vi "HMI.vi"(8 "error in (no error)":errorcluster caption="entrée d'erreur (pas d'erreur)", 11 "Class Popup Autotest (Default) en entrée":refnum<class "Popup Autotest_With_Actor.lvclass">) -> (0 "error out":errorcluster caption="sortie d'erreur", 1 "Input":string, 2 "Autotest":bool, 3 "Class Popup Autotest (Default) en sortie":refnum<class "Popup Autotest_With_Actor.lvclass">)   [LabVIEW 2020, in "Library Instrument & Equipement.lvlib" / "Library Popup.lvlib" / "Popup Autotest_With_Actor.lvclass"]
uses:
  Popup Autotest_With_Actor.lvclass
  C:/Users/ngarcin/OneDrive - Altyor/Standard TB/Class/Popup/Class Popup (Main)/Class Popup (Main).lvclass
  C:/Users/ngarcin/OneDrive - Altyor/Standard TB/Class/Popup/Class Popup Autotest (Default)/Popup Autotest (Default).lvclass
  Commun VI/TypeDef/Commande Popup autotest/Commande element autotest.ctl
  Instrument/Instrument (Default)/Class Instrument (Default).lvclass
  Core/Actors/Actor_Autotest/Auto-test/Auto-test/Actor_Autotest.lvclass
  C:/Program Files (x86)/National Instruments/LabVIEW 2020/vi.lib/ActorFramework/Actor/Actor.lvclass
  Core/Actors/Actor_Autotest/Auto-test/Actor_Autotest Messages/Load_Instr_Object Msg/Load_Instr_Object Msg.lvclass/Load_Instr_Object Msg.ctl
  <vilib>/ActorFramework/Message Enqueuer/Message Enqueuer.lvclass/Message Enqueuer.ctl
  <vilib>/ActorFramework/Stop Msg/Stop Msg.lvclass/Stop Msg.ctl
  <vilib>/ActorFramework/Message Enqueuer/Enqueue.vi
  <vilib>/ActorFramework/Message Enqueuer/Enqueue Critical.vi
  Core/Actors/Actor_Autotest/Auto-test/Actor_Autotest Messages/Load_Instr_Object Msg/Load_Instr_Object Msg.lvclass
  C:/Program Files (x86)/National Instruments/LabVIEW 2020/vi.lib/ActorFramework/Message/Message.lvclass
  Core/Actors/Actor_Autotest/Auto-test/Actor_Autotest Messages/Register_Actor Msg/Register_Actor Msg.lvclass
  <vilib>/ActorFramework/Stop Msg/Stop Msg.lvclass
  <vilib>/ActorFramework/Message Priority Queue/Priority Enqueue.vi
  Variable Instr.vi
  <vilib>/regexp/Match Regular Expression.xnode
  Class Popup Autotest (Default)/Popup Autotest (Default).lvclass
  Popup Autotest_With_Actor.lvclass/Popup Autotest_With_Actor.ctl
  <vilib>/ActorFramework/Actor/Actor.lvclass
  Commun VI/Library Commun.lvlib
panel:
  out "Element test":T2
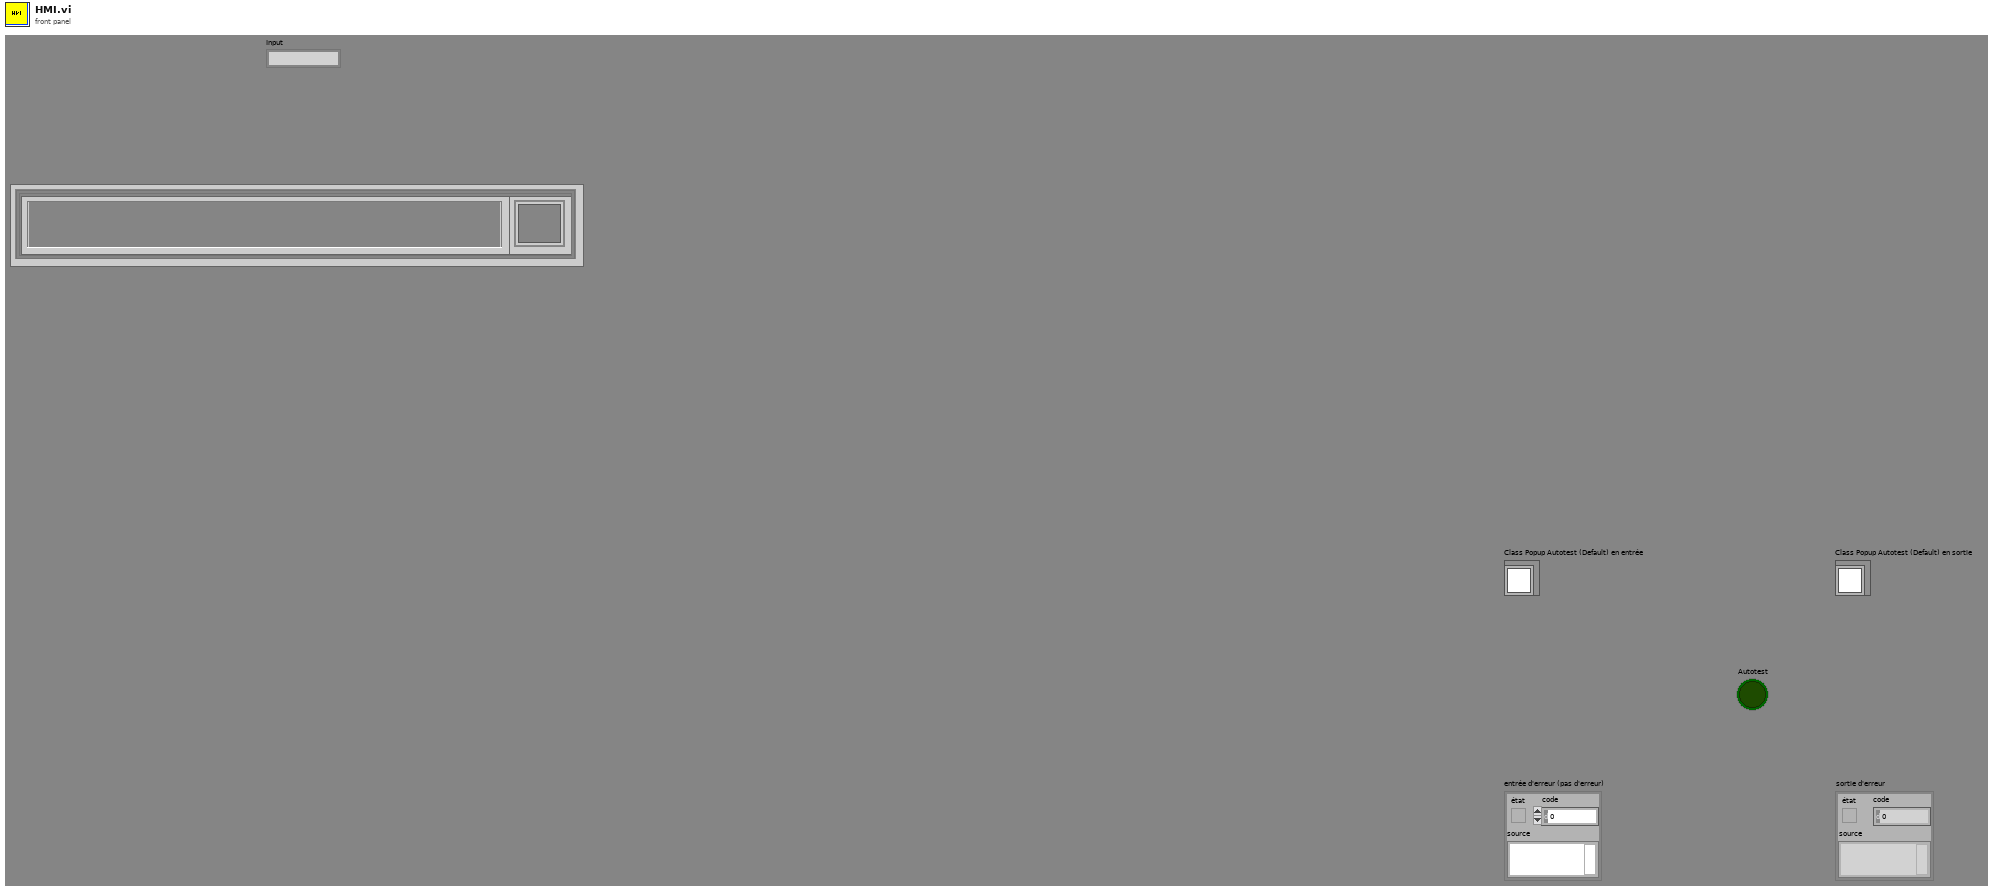
[diagram p1: front panel]
types:
  T1 = typedef "Commande element autotest.ctl" = cluster{"Instrument":string, "Etat":cluster{"Menu déroulant":u16}}
  T2 = cluster{"Element autotest":T1, "Element autotest 2":T1, "Element autotest 3":T1, "Element autotest 4":T1, "Element autotest 5":T1, "Element autotest 6":T1, "Element autotest 7":T1, "Element autotest 8":T1, "Element autotest 9":T1}
  T3 = cluster{"Instrument":refnum<class "Class Instrument (Default).lvclass">, "Element autotest":T1}
  T4 = cluster{"Name":string, "Instrument":refnum<class "Class Instrument (Default).lvclass">, "Close After Autotest":bool}[]
  T5 = enum16{"Init", "Add Actor", "Delete Actor", "Get Actor Queue", "Get Log Actor Queue", "List all actors"}
  T6 = cluster{"Name":string, "Instrument":refnum<class "Class Instrument (Default).lvclass">, "Close After Autotest":bool}
  T7 = cluster{"[0]":T1, "[1]":T1, "[2]":T1, "[3]":T1, "[4]":T1, "[5]":T1, "[6]":T1, "[7]":T1, "[8]":T1}
  T8 = typedef "LVRectTypeDef.ctl" = cluster{"Left":i16, "Top":i16, "Right":i16, "Bottom":i16}
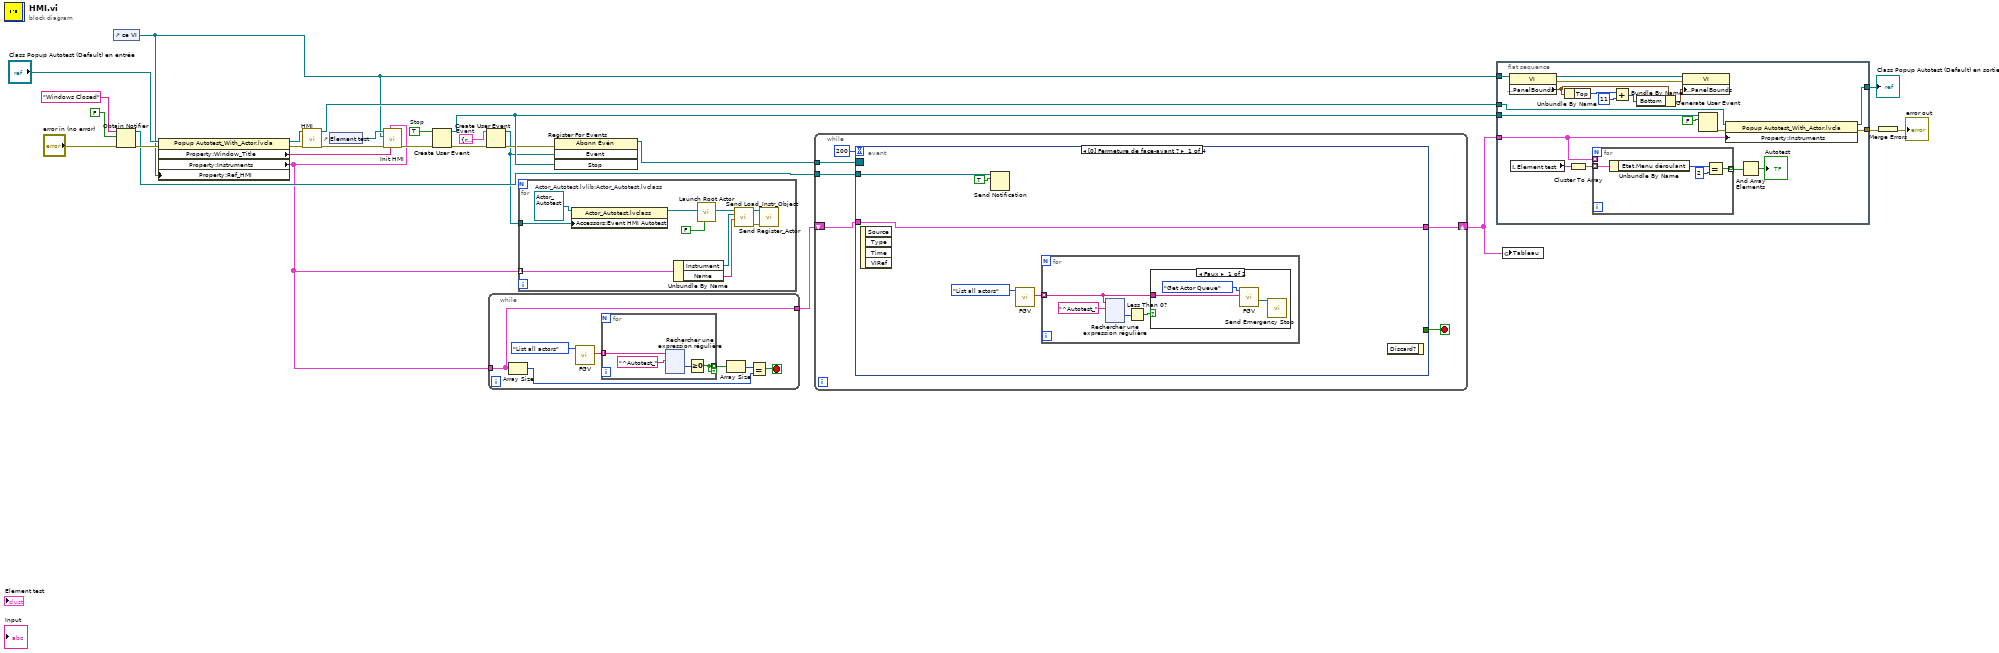
[diagram p0: block diagram]
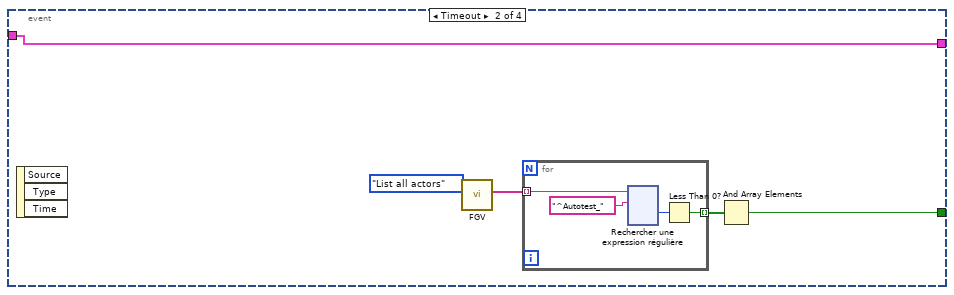
[diagram p3: hidden frame]
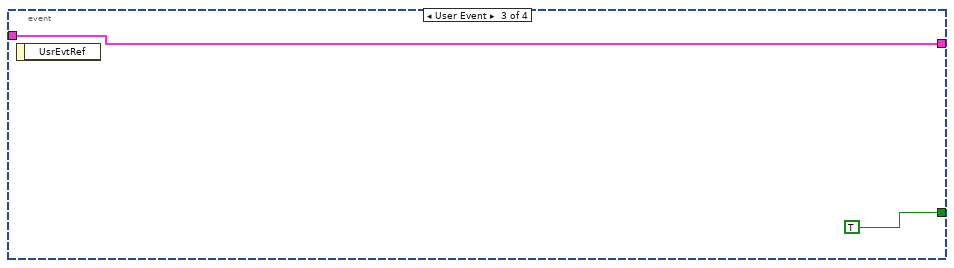
[diagram p4: hidden frame]
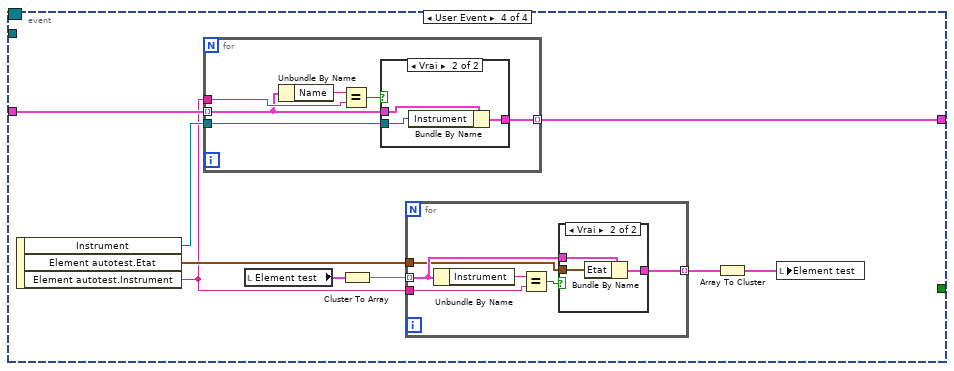
[diagram p5: hidden frame]
diagram:
  w4 = T3 {"Instrument"=refnum, "Element autotest"={"Instrument"="", "Etat"={"Menu déroulant"=0}}}  # Event
  w14 = TRUE  # Stop
  n1 = control-ref of="ce VI"() -> (w8:refnum<vi>)
  n2 = Obtain Notifier(name (unnamed)="Windows Closed" ("nom (aucun)"), notification data type=FALSE, error in (no error)="error in (no error)") -> (notifier out=w16:refnum<notifier>, error out=w19:errorcluster)  [unwired: 1 in, 1 out]
  n3 = property class="Popup Autotest_With_Actor.lvcla"(reference="Class Popup Autotest (Default) en entrée", error in=w19, "Property:Ref_HMI"=w8) -> (reference out=w27:refnum<class "Popup Autotest_With_Actor.lvclass">, error out=w9:errorcluster, "Property:Window_Title"=w24:string, "Property:Instruments"=w3:T4)
  n4 = call-parent "HMI.vi"("error in (no error)"=w9, "Class Popup Autotest (Default) en entrée"=w27) -> ("error out"=w23:errorcluster, "Class Popup Autotest (Default) en sortie"=w20:refnum<class "Popup Autotest_With_Actor.lvclass">)  [unwired: 6 in, 2 out]
  n5 = control-ref of="Element test"() -> (w25:refnum<vi>)
  n6 = call "Init HMI.vi"("Window_Title"=w24, "Instruments"=w3, "entrée d'erreur (pas d'erreur)"=w23, "ce VI"=w8, "Cluster en entrée"=w25) -> ("sortie d'erreur"=w13:errorcluster)  [unwired: 5 in, 1 out]
  n7 = Create User Event(user event datatype=w14, error in=w13) -> (user event=w12:refnum<user-event>, error out=w7:errorcluster)
  n8 = Create User Event(user event datatype=w4, error in=w7) -> (user event=w5:refnum<user-event>, error out=w6:errorcluster)
  n9 = while {
    tunnel: w3 -> [w32]
    tunnel: [w32] -> w2
    stop <- w33 stop-if-true
    n10 = Array Size(array=w32) -> (size(s)=w28:i32)
    n11 = call "FGV.vi"("Action"=T5."List all actors") -> ("Actor names"=w31:string[])  [unwired: 8 in, 2 out]
    n12 = for {
      tunnel: w31 -> [w38] mode=indexing
      tunnel: [w35] -> w30 mode=indexing if=w35
      n13 = xnode "Rechercher une expression régulière"("chaîne en entrée"=w38, "expression régulière"="^Autotest_" ("élément")) -> ("offset après correspondance"=w36:i32)  [unwired: 4 in, 4 out]
      n14 = Greater Or Equal To 0?(x=w36) -> (x >= 0?=w35:bool)
    }
    n15 = Array Size(array=w30) -> (size(s)=w29:i32)
    n16 = Equal?(x=w29, y=w28) -> (x = y?=w33:bool)
  }
  n17 = for {
    tunnel: w5 -> [w160]
    tunnel: w3 -> [w157] mode=indexing
    w161 = refnum<class "Actor_Autotest.lvclass"> refnum  # Actor_Autotest.lvlib:Actor_Autotest.lvclass
    n18 = property class="Actor_Autotest.lvclass"(reference=w161, "Accessors:Event HMI Autotest"=w160) -> (reference out=w159:refnum<class "Actor_Autotest.lvclass">)  [unwired: 1 in, 1 out]
    n19 = Unbundle By Name(w157) -> ("Instrument"=w156:refnum<class "Class Instrument (Default).lvclass">, "Name"=w155:string)
    n20 = call <vilib>:"Launch Root Actor.vi"("Open Actor Core front panel? (F)"=FALSE, "Actor"=w159) -> ("Actor's Enqueuer"=w158:refnum<class "Message Enqueuer.lvclass">)  [unwired: 8 in, 1 out]
    n21 = call "Send Load_Instr_Object.vi"("Instr name"=w155, "Instr obj"=w156, "Message Enqueuer"=w158) -> ("error out"=w153:errorcluster, "Message Enqueuer out"=w154:refnum<class "Message Enqueuer.lvclass">)  [unwired: 7 in]
    n22 = call "Send Register_Actor.vi"("error in (no error)"=w153, "Message Enqueuer"=w154) -> ()  [unwired: 8 in, 2 out]
  }
  n23 = register-events(error in=w6, w5, w12) -> (reference out=w15:refnum<event-registration>)  [unwired: 1 in, 1 out]
  n24 = while {
    tunnel: w16 -> [w168]
    tunnel: w15 -> [w167]
    shift-right: [w164] -> w1
    shift-left: w2 -> [w165]
    stop <- w166 stop-if-true
    n25 = event shown="[0] Fermeture de face-avant ?" {
      selector: w167 -> [_ _ _ _]
      dyn-events: _ -> [_ _ _ _]
      timeout: 200 -> [_ _ _ _]
      tunnel: w168 -> [w173 _ _ _]
      tunnel: [_ w296 TRUE _] -> w166
      tunnel: w165 -> [w171 w295 w418 w423]
      tunnel: [w171 w295 w418 w422] -> w164
      event Panel Close? {
        n26 = event-data() -> ()  [unwired: 1 in, 4 out]
        n27 = Send Notification(notification=TRUE, notifier=w173) -> ()  [unwired: 1 in, 2 out]
        n28 = call "FGV.vi"("Action"=T5."List all actors") -> ("Actor names"=w169:string[])  [unwired: 8 in, 2 out]
        n29 = for {
          tunnel: w169 -> [w174] mode=indexing
          n30 = xnode "Rechercher une expression régulière"("chaîne en entrée"=w174, "expression régulière"="^Autotest_" ("élément")) -> ("offset après correspondance"=w176:i32)  [unwired: 4 in, 4 out]
          n31 = Less Than 0?(x=w176) -> (x < 0?=w175:bool)
          n32 = case shown="Faux" w175 {
            tunnel: w174 -> [w179 _]
            frame False {
              n33 = call "FGV.vi"("Actor name"=w179, "Action"=T5."Get Actor Queue") -> ("Actor's Queue Out"=w178:refnum<class "Message Enqueuer.lvclass">)  [unwired: 7 in, 2 out]
              n34 = call <vilib>:"Send Emergency Stop.vi"("Message Enqueuer"=w178) -> ()  [unwired: 10 in, 1 out]
            }
            frame True {
            }
          }
        }
        n35 = event-data() -> ()  [unwired: 2 in, 1 out]
      }
      event Timeout {
        n36 = event-data() -> ()  [unwired: 1 in, 3 out]
        n37 = call "FGV.vi"("Action"=T5."List all actors") -> ("Actor names"=w298:string[])  [unwired: 8 in, 2 out]
        n38 = for {
          tunnel: w298 -> [w303] mode=indexing
          tunnel: [w300] -> w297 mode=indexing
          n39 = xnode "Rechercher une expression régulière"("chaîne en entrée"=w303, "expression régulière"="^Autotest_" ("élément")) -> ("offset après correspondance"=w301:i32)  [unwired: 4 in, 4 out]
          n40 = Less Than 0?(x=w301) -> (x < 0?=w300:bool)
        }
        n41 = And Array Elements(Boolean array=w297) -> (logical AND=w296:bool)
      }
      event User Event {
        n42 = event-data() -> ()  [unwired: 1 in, 1 out]
      }
      event User Event {
        n43 = event-data() -> ("Instrument"=w421:refnum<class "Class Instrument (Default).lvclass">, "Element autotest.Etat"=w427:cluster{"Menu déroulant":u16}, "Element autotest.Instrument"=w420:string)  [unwired: 1 in]
        n44 = for {
          tunnel: w423 -> [w430] mode=indexing
          tunnel: w420 -> [w433]
          tunnel: w421 -> [w431]
          tunnel: [w429] -> w422 mode=indexing
          n45 = Unbundle By Name(w430) -> ("Name"=w434:string)
          n46 = Equal?(x=w434, y=w433) -> (x = y?=w432:bool)
          n47 = case shown="Vrai" w432 {
            tunnel: w431 -> [_ w437]
            tunnel: w430 -> [w435 w438]
            tunnel: [w435 w436] -> w429
            frame False {
            }
            frame True {
              n48 = Bundle By Name(cluster=w438, "Instrument"=w437) -> (w436:T6)
            }
          }
        }
        n49 = local read "Element test"() -> (w425:T2)
        n50 = Cluster To Array(cluster=w425) -> (array=w428:T1[])
        n51 = for {
          tunnel: w428 -> [w441] mode=indexing
          tunnel: w420 -> [w444]
          tunnel: w427 -> [w440]
          tunnel: [w439] -> w426 mode=indexing
          n52 = Unbundle By Name(w441) -> ("Instrument"=w443:string)
          n53 = Equal?(x=w443, y=w444) -> (x = y?=w442:bool)
          n54 = case shown="Vrai" w442 {
            tunnel: w441 -> [w445 w448]
            tunnel: w440 -> [_ w447]
            tunnel: [w445 w446] -> w439
            frame False {
            }
            frame True {
              n55 = Bundle By Name(cluster=w448, "Etat"=w447) -> (w446:T1)
            }
          }
        }
        n56 = Array To Cluster(array=w426) -> (cluster=w424:T7)
        n57 = local write "Element test"(w424) -> ()
      }
    }
  }
  n58 = flat-sequence {
    tunnel: [w467] -> w22
    tunnel: w20 -> [w466]
    tunnel: w12 -> [w464]
    tunnel: [w462] -> w11
    tunnel: w8 -> [w454]
    tunnel: w1 -> [w449]
    frame #0 {
      n59 = property class="VI"(reference=w454) -> (reference out=w459:refnum<vi>, error out=w461:errorcluster, "Front Panel.PanelBounds"=w460:T8)  [unwired: 1 in]
      n60 = local read "Element test"() -> (w453:T2)
      n61 = Unbundle By Name(w460) -> ("Top"=w458:i16)
      n62 = Cluster To Array(cluster=w453) -> (array=w452:T1[])
      n63 = for {
        tunnel: w452 -> [w471] mode=indexing
        tunnel: [w468] -> w451 mode=indexing
        tunnel: w449 -> [_] mode=indexing
        n64 = Unbundle By Name(w471) -> ("Etat.Menu déroulant"=w470:u16)
        n65 = Equal?(x=w470, y=u16 2) -> (x = y?=w468:bool)
      }
      n66 = Add(x=w458, y=i16 11) -> (x+y=w457:i16)
      n67 = Bundle By Name(cluster=w460, "Bottom"=w457) -> (w456:T8)
      n68 = property class="VI"(reference=w459, error in=w461, "Front Panel.PanelBounds"=w456) -> ()  [unwired: 2 out]
      n69 = Generate User Event(user event=w464, event data cluster=FALSE ("données d'événement")) -> (error out=w465:errorcluster)  [unwired: 2 in, 1 out]
      n70 = property class="Popup Autotest_With_Actor.lvcla"(reference=w466, error in=w465, "Property:Instruments"=w449) -> (reference out=w467:refnum<class "Popup Autotest_With_Actor.lvclass">, error out=w462:errorcluster)
      n71 = And Array Elements(Boolean array=w451) -> (logical AND=→"Autotest":bool)
    }
  }
  n72 = global write "Variable Instr.vi" "Tableau"(w1) -> ()
  n73 = Merge Errors(w11) -> (→"error out":errorcluster)
  "Class Popup Autotest (Default) en sortie" <- w22
